vi "Set_AO.vi"(8 "error in (no error)":errorcluster, 9 "PWM":i8, 10 "PIN":i8, 11 "Driver_AI_AO in":refnum<class "Driver_AI_AO.lvclass">) -> (0 "error out":errorcluster, 3 "Driver_AI_AO out":refnum<class "Driver_AI_AO.lvclass">)   [LabVIEW 2023, in "Driver_AI_AO.lvlib" / "Driver_AI_AO.lvclass"]
uses:
  Driver_AI_AO.lvclass
  Driver_AI_AO.lvclass/Driver_AI_AO.ctl
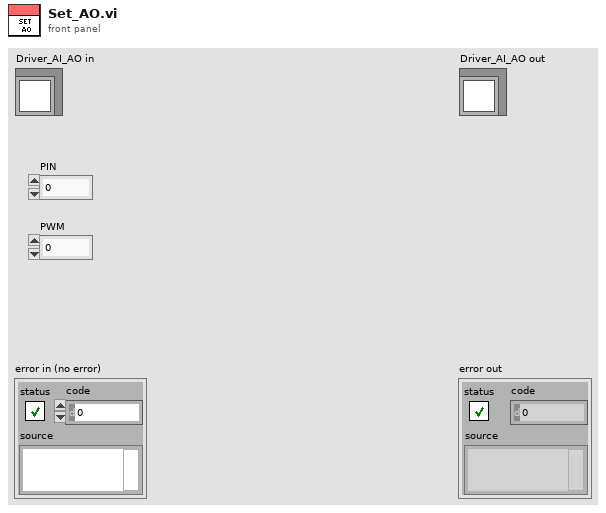
[diagram p1: front panel]
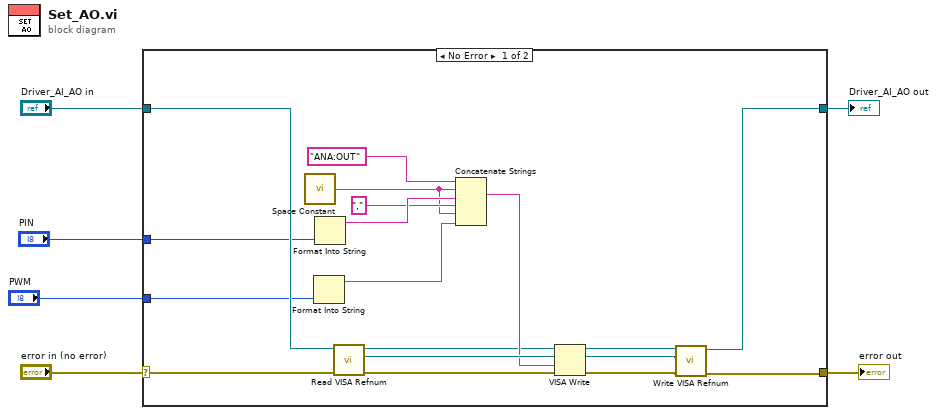
[diagram p0: block diagram]
diagram:
  n1 = case shown="No Error" "error in (no error)" {
    selector: "error in (no error)" -> [w13 w25]
    tunnel: [w12 w25] -> w5
    tunnel: [w11 w24] -> w3
    tunnel: "Driver_AI_AO in" -> [w10 w24]
    tunnel: "PIN" -> [w9 _]
    tunnel: "PWM" -> [w8 _]
    frame No Error {
      n2 = call <vilib>:"Space Constant.vi"() -> ("String"=w14:string)
      n3 = Format Into String(w8) -> (resulting string=w7:string)  [unwired: 3 in, 1 out]
      n4 = Format Into String(w9) -> (resulting string=w20:string)  [unwired: 3 in, 1 out]
      n5 = call-dynamic "Read VISA Refnum.vi"("error in (no error)"=w13, "Driver in"=w10) -> ("error out"=w23:errorcluster, "VISA Refnum"=w22:refnum<visa-resource-name>, "Driver out"=w16:refnum<class "Driver_AI_AO.lvclass">)  [unwired: 7 in]
      n6 = Concatenate Strings("ANA:OUT" ("string"), w14, w20, ",", w14, w7) -> (w19:string)
      n7 = VISA Write(VISA resource name=w22, write buffer=w19, error in (no error)=w23) -> (VISA resource name out=w17:refnum<visa-resource-name>, error out=w18:errorcluster)  [unwired: 1 out]
      n8 = call-dynamic "Write VISA Refnum.vi"("error in (no error)"=w18, "VISA Refnum"=w17, "Driver in"=w16) -> ("error out"=w12:errorcluster, "Driver out"=w11:refnum<class "Driver_AI_AO.lvclass">)  [unwired: 7 in]
    }
    frame Error {
    }
  }
  "error out" <- w5
  "Driver_AI_AO out" <- w3
